vi "UpdateTree(MultipleLines).vi"(8 "error in (no error)":errorcluster, 10 "SR Data":string[][](array[string]), 11 "Tree Reference In":refnum<vi>) -> (0 "error out":errorcluster, 3 "Tree Reference Out":refnum<vi>)   [LabVIEW 2017, in "Client.lvlib" / "UI_API.lvlib"]
uses:
  UI_API.lvlib
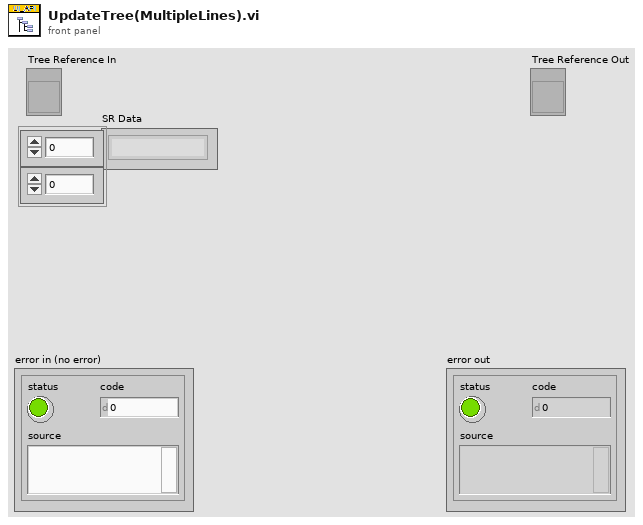
[diagram p1: front panel]
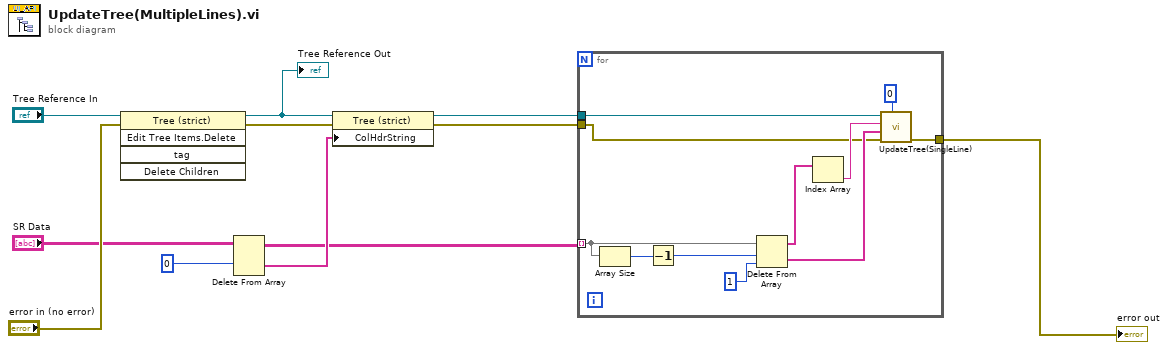
[diagram p0: block diagram]
diagram:
  n1 = invoke on="Invoke Node" class="Tree (strict)" method="Edit Tree Items.Delete"(reference="Tree Reference In", error in="error in (no error)") -> (reference out=w5:refnum<vi>, error out=w6:errorcluster)  [unwired: 3 in, 3 out]
  "Tree Reference Out" <- w5
  n2 = Delete From Array(array="SR Data", index (row)=0) -> (deleted portion=w2:string[], array with subset deleted=w1:string[][])  [unwired: 2 in]
  n3 = property class="Tree (strict)"(reference=w5, error in=w6, "ColHdrString"=w2) -> (reference out=w8:refnum<vi>, error out=w7:errorcluster)
  n4 = for {
    tunnel: w8 -> [w22]
    tunnel: w1 -> [w18] mode=indexing
    tunnel: w7 -> [w13]
    tunnel: [w12] -> w9
    n5 = Array Size(array=w18) -> (size(s)=w17:i32)
    n6 = Decrement(x=w17) -> (x-1=w16:i32)
    n7 = Delete From Array(array=w18, length=w16, index=1) -> (deleted portion=w15:string[], array with subset deleted=w20:string[])
    n8 = Index Array(array=w20) -> (element=w19:string)  [unwired: 1 in]
    n9 = call "UpdateTree(SingleLine).vi"("New Item Indentation"=0, "error in (no error)"=w13, "Item Properties"=w15, "Item Name"=w19, "Tree Reference"=w22) -> ("error out"=w12:errorcluster)  [unwired: 6 in]
  }
  "error out" <- w9
